vi "ungerade.vi"(11 "Zahl":u32) -> (3 "ungerade ?":bool)   [LabVIEW 2020, in "Linearisierung v2.lvlib" / "SpanEinstellungen.lvlib"]
uses:
  SpanEinstellungen.lvlib
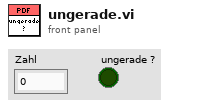
[diagram p1: front panel]
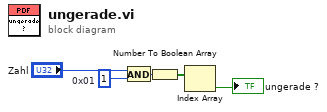
[diagram p0: block diagram]
diagram:
  w4 = u32 1  # 0x01
  n1 = And(x="Zahl", y=w4) -> (x .and. y?=w3:u32)
  n2 = Number To Boolean Array(number=w3) -> (Boolean array=w2:bool[])
  n3 = Index Array(array=w2) -> (element=→"ungerade ?":bool)  [unwired: 1 in]
